vi "SO2 TCP Packet_v3.vi"(7 "TCP Packet In":string, 13 "Data Array":string[](array[string])) -> (8 "TCP Binary Packet":string)   [LabVIEW 2014]
panel:
  out "array":string[](array[string])
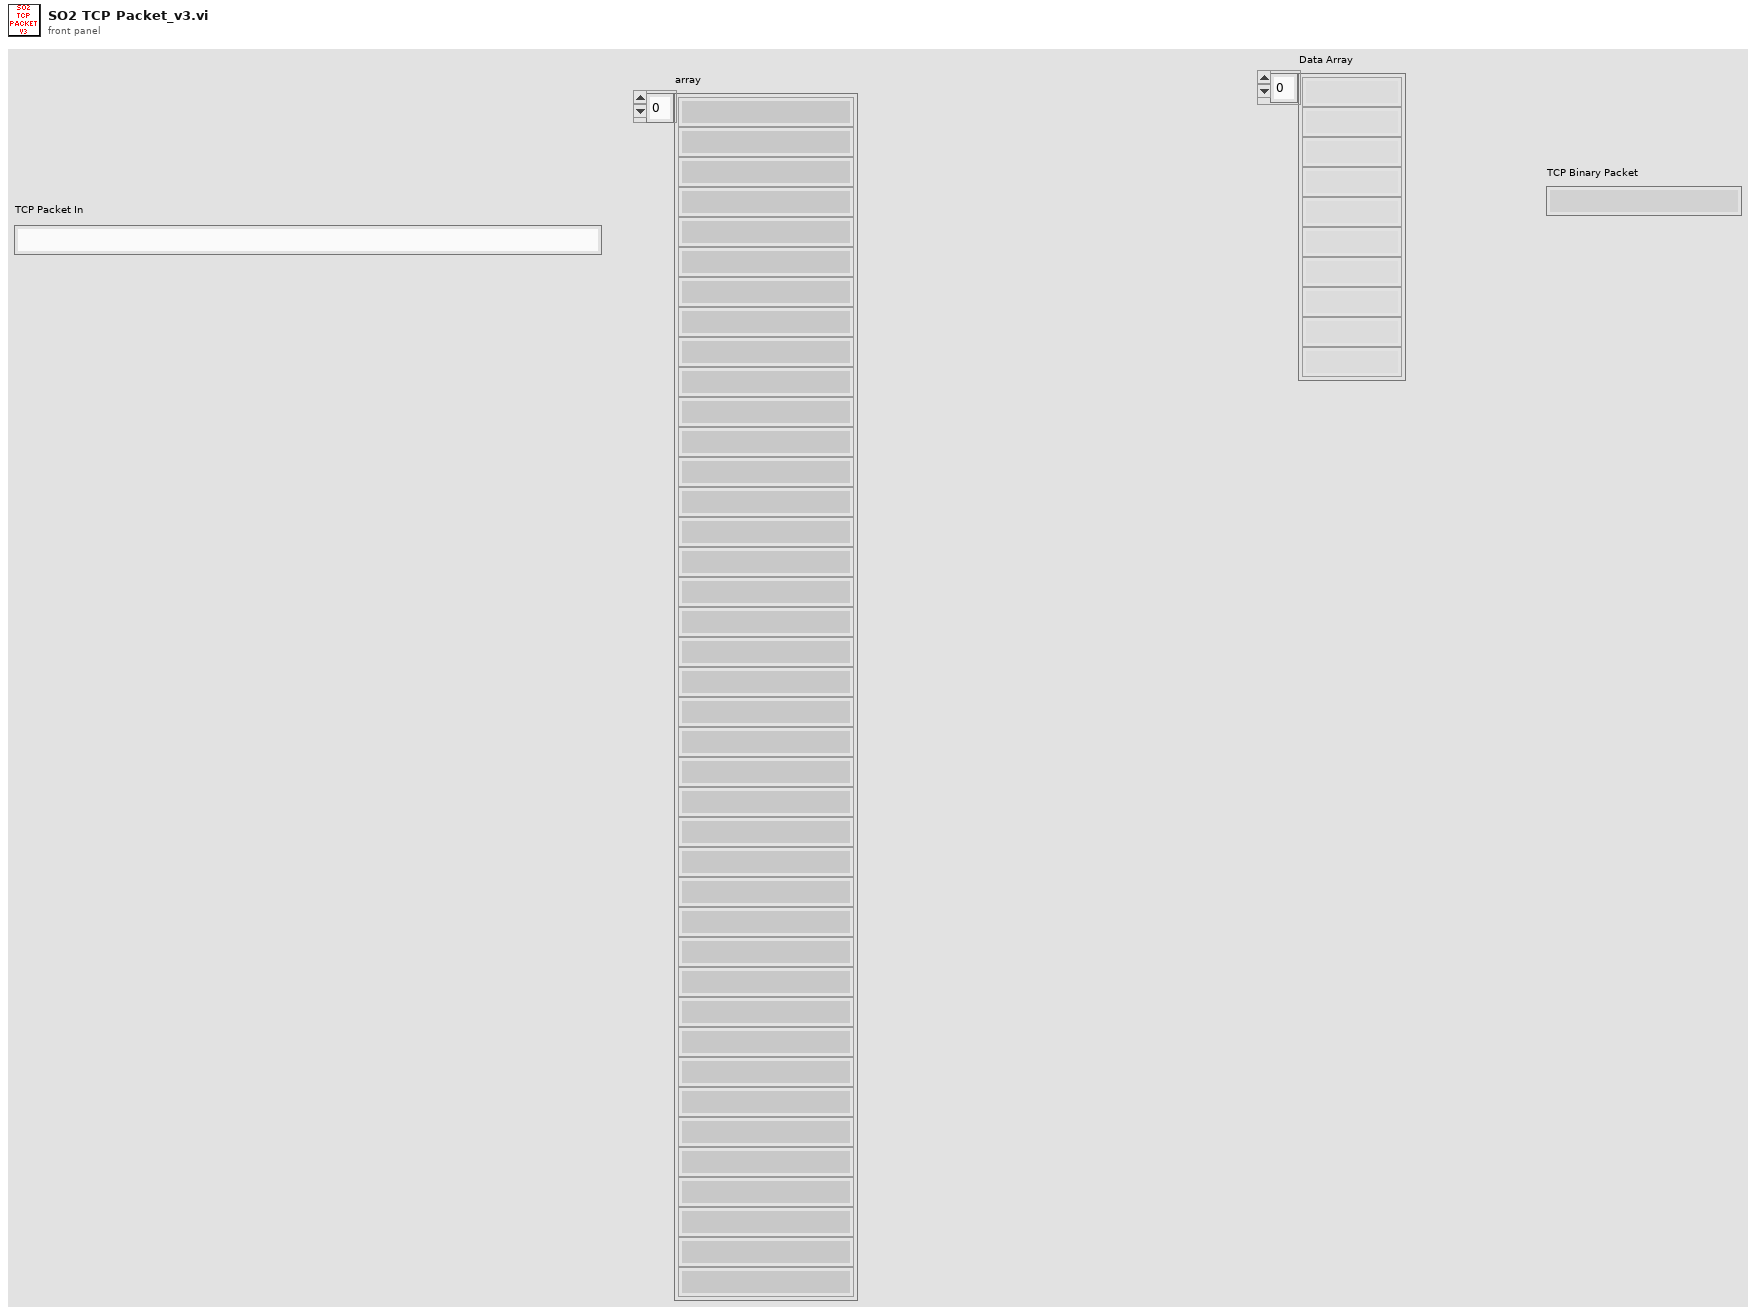
[diagram p1: front panel]
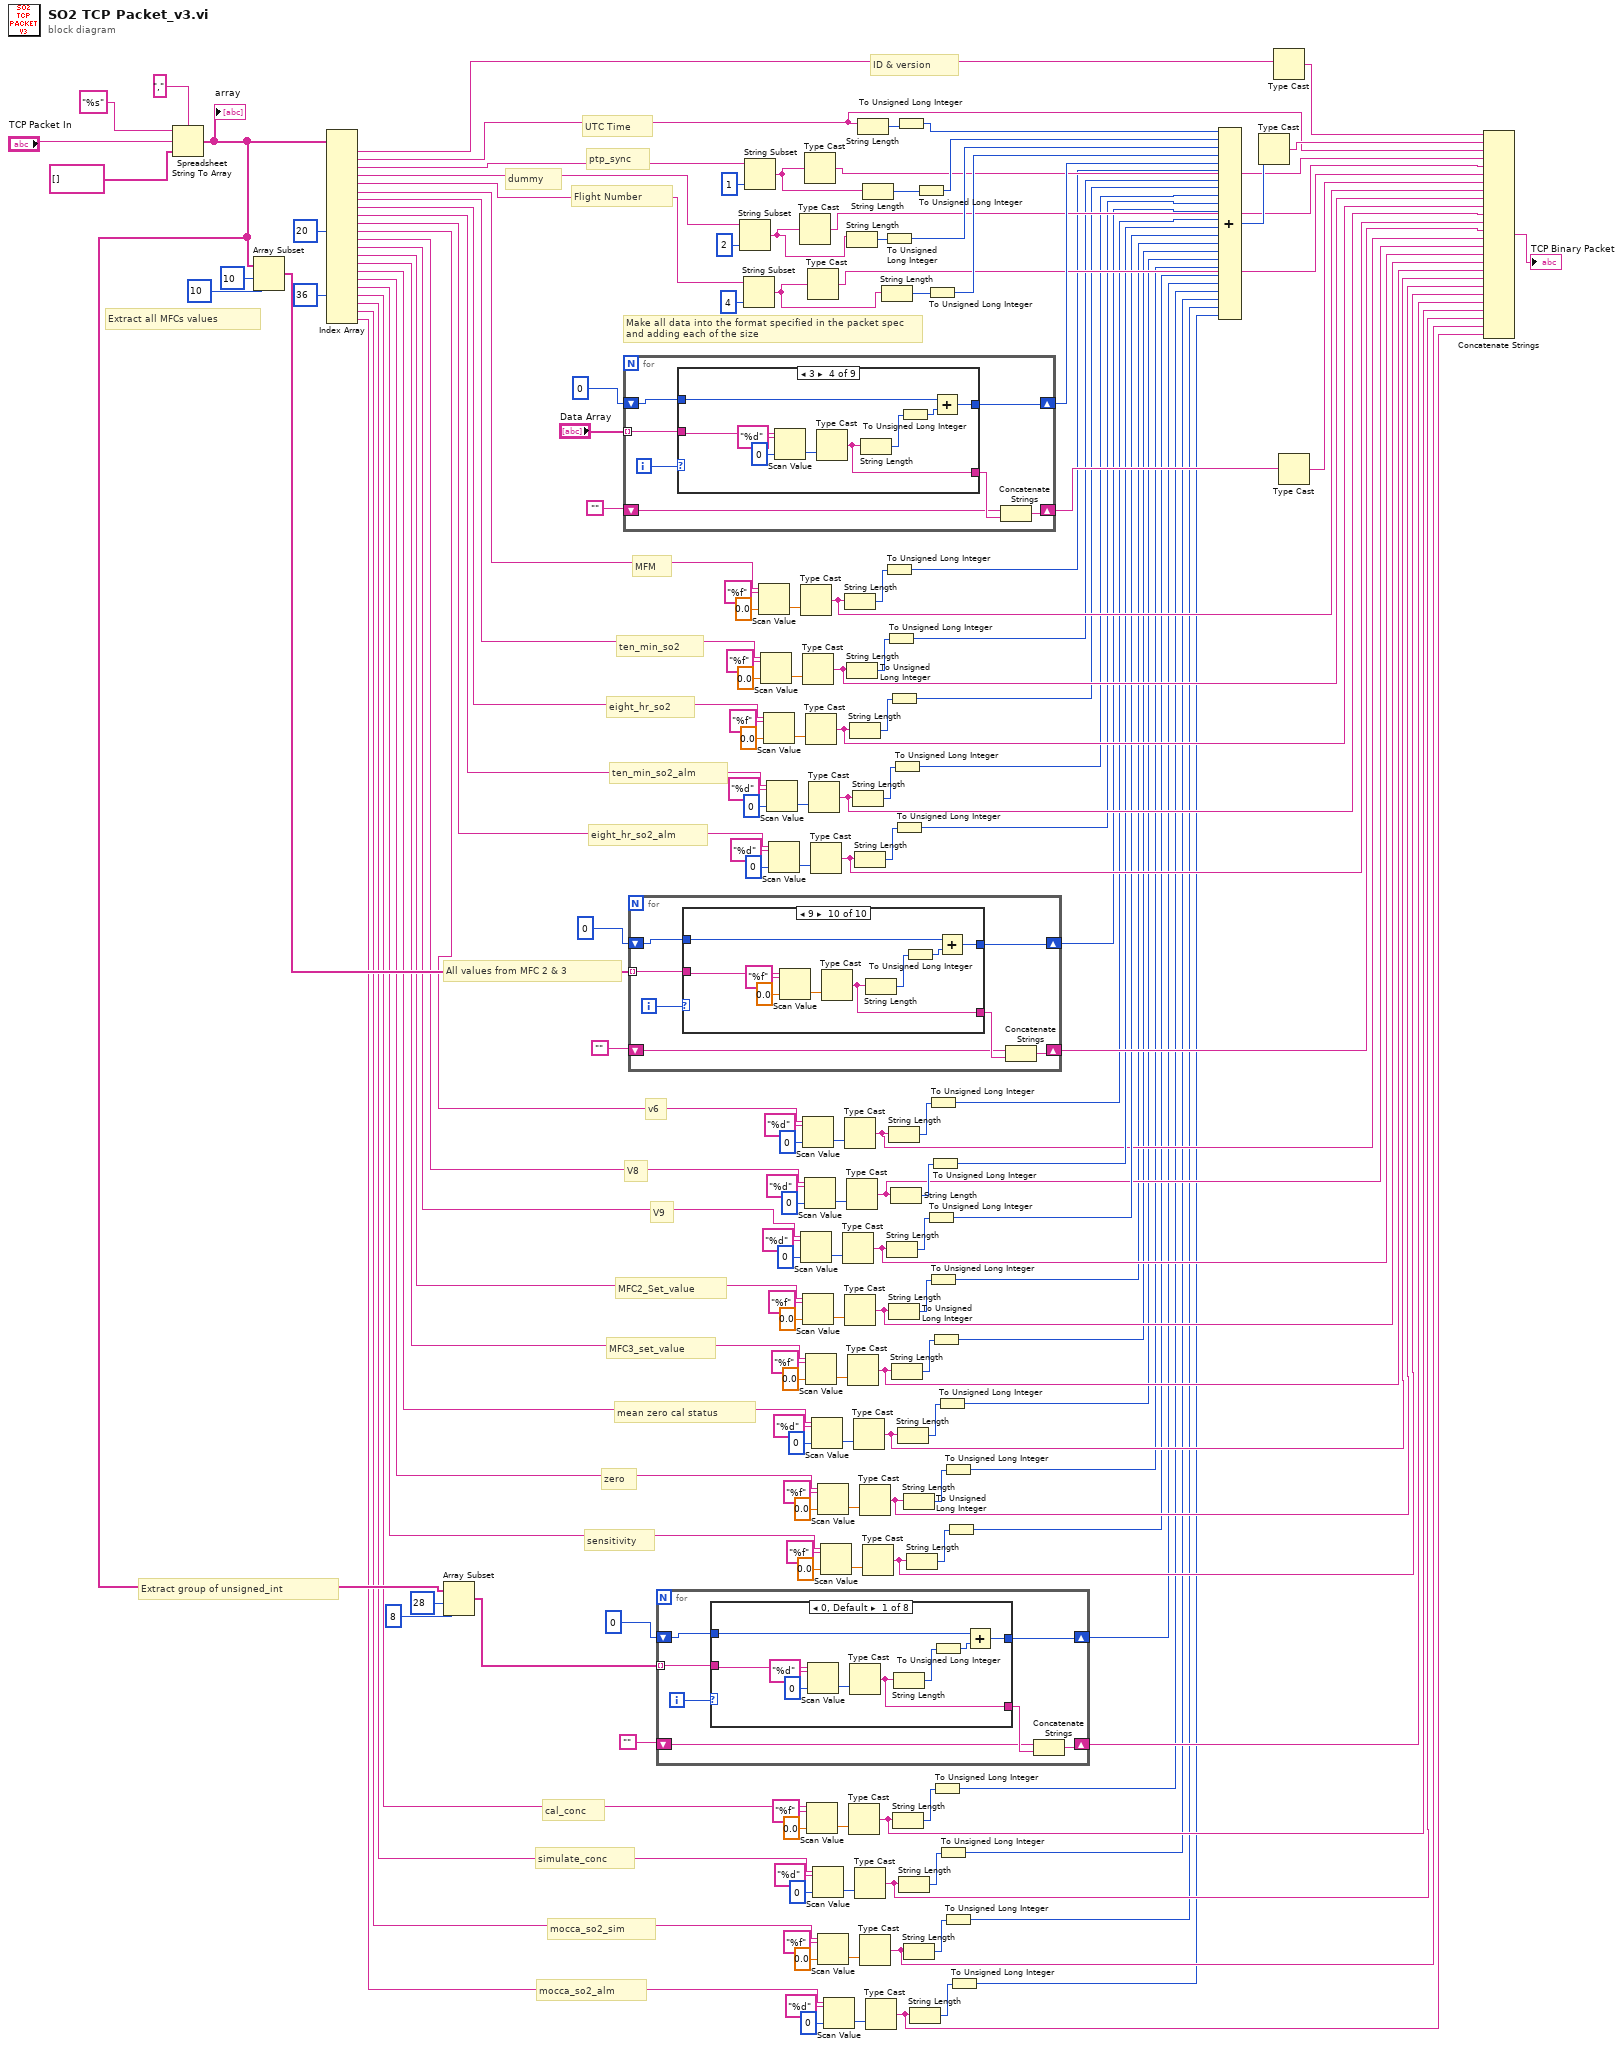
[diagram p0: block diagram]
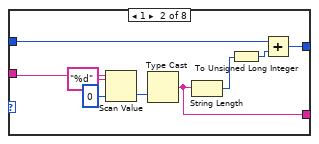
[diagram p2: hidden frame]
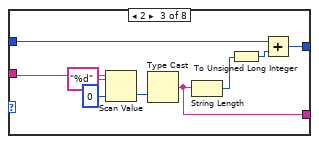
[diagram p3: hidden frame]
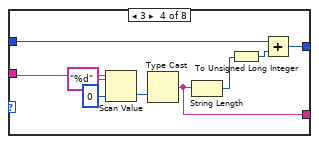
[diagram p4: hidden frame]
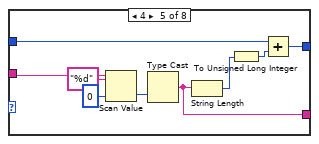
[diagram p5: hidden frame]
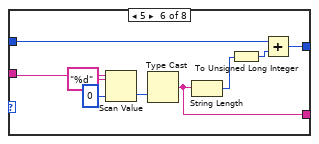
[diagram p6: hidden frame]
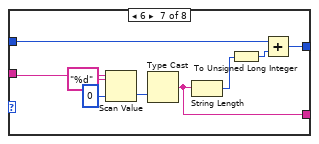
[diagram p7: hidden frame]
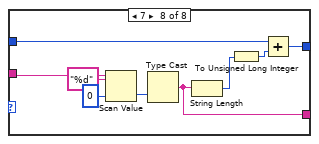
[diagram p8: hidden frame]
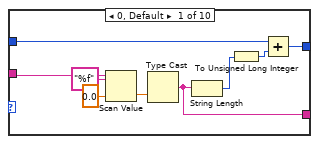
[diagram p9: hidden frame]
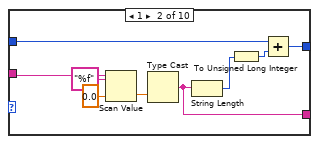
[diagram p10: hidden frame]
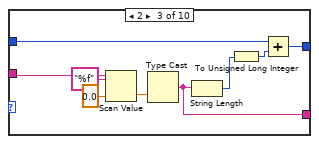
[diagram p11: hidden frame]
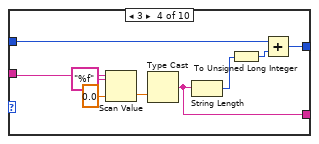
[diagram p12: hidden frame]
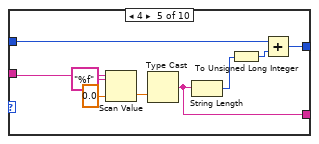
[diagram p13: hidden frame]
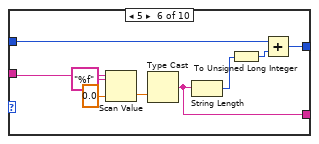
[diagram p14: hidden frame]
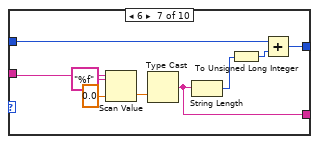
[diagram p15: hidden frame]
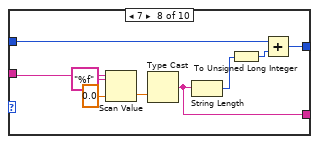
[diagram p16: hidden frame]
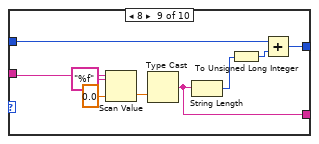
[diagram p17: hidden frame]
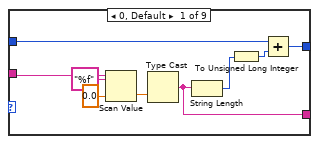
[diagram p18: hidden frame]
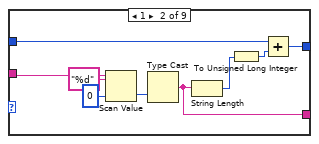
[diagram p19: hidden frame]
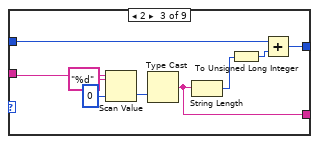
[diagram p20: hidden frame]
diagram:
  # "mocca_so2_alm"
  # "mocca_so2_sim"
  # "simulate_conc"
  # "cal_conc"
  # "Extract group of unsigned_int"
  # "sensitivity"
  # "zero"
  # "mean zero cal status"
  # "MFC3_set_value"
  # "MFC2_Set_value"
  # "V9"
  # "V8"
  # "v6"
  # "All values from MFC 2 & 3"
  # "Extract all MFCs values"
  # "eight_hr_so2_alm"
  # "ten_min_so2_alm"
  # "eight_hr_so2"
  # "ten_min_so2"
  # "MFM"
  # "Flight Number"
  # "dummy"
  # "ptp_sync"
  # "UTC Time"
  # "ID & version"
  # "Make all data into the format specified in the packet spec\nand adding each of the size"
  n1 = Spreadsheet String To Array(delimiter (Tab)=",", format string="%s", spreadsheet string="TCP Packet In", array type (2D Dbl)=string[] []) -> (array=w35:string[])
  "array" <- w35
  n2 = Array Subset(array=w35, index=10, length=10) -> (w97:string[])
  n3 = Index Array(array=w35, index #11=20 ("index"), index #19=36 ("index")) -> (element #1=w141:string, element #2=w140:string, element #3=w139:string, element #4=w138:string, element #5=w137:string, element #6=w132:string, element #7=w121:string, element #8=w118:string, element #9=w107:string, element #10=w104:string, element #11=w85:string, element #12=w84:string, element #13=w79:string, element #14=w64:string, element #15=w59:string, element #16=w54:string, element #17=w43:string, element #18=w38:string, element #19=w12:string, element #20=w3:string, element #21=w2:string, element #22=w1:string)  [unwired: 20 in]
  n4 = Array Subset(array=w35, index=28, length=8) -> (w31:string[])
  n5 = for {
    tunnel: "Data Array" -> [w178] mode=indexing
    shift-right: [w176] -> w160
    shift-left: u32 0 -> [w177]
    shift-right: [w175] -> w149
    shift-left: "" -> [w173]
    i -> [w179]
    n6 = case shown="3" w179 {
      tunnel: w178 -> [w186 w195 w204 w213 w222 w231 w240 w249 w253]
      tunnel: w177 -> [w184 w193 w202 w211 w220 w229 w238 w247 w259]
      tunnel: [w181 w190 w199 w208 w217 w226 w235 w244 w256] -> w176
      tunnel: [w180 w189 w198 w207 w216 w225 w234 w243 w255] -> w174
      frame 0, Default {
        n7 = Scan Value(string=w186, format string="%f", default (0 dbl)=sgl 0.0 ("default (0 I32)")) -> (value=w188:sgl)  [unwired: 1 out]
        n8 = Type Cast(x=w188) -> (*(type *) &x=w180:string)  [unwired: 1 in]
        n9 = String Length(string=w180) -> (length=w183:i32)
        n10 = To Unsigned Long Integer(number=w183) -> (unsigned 32bit integer=w182:u32)
        n11 = Add(x=w184, y=w182) -> (x+y=w181:u32)
      }
      frame 1 {
        n12 = Scan Value(string=w195, format string="%d", default (0 dbl)=0 ("default (0 I32)")) -> (value=w197:i32)  [unwired: 1 out]
        n13 = Type Cast(x=w197) -> (*(type *) &x=w189:string)  [unwired: 1 in]
        n14 = String Length(string=w189) -> (length=w192:i32)
        n15 = To Unsigned Long Integer(number=w192) -> (unsigned 32bit integer=w191:u32)
        n16 = Add(x=w193, y=w191) -> (x+y=w190:u32)
      }
      frame 2 {
        n17 = Scan Value(string=w204, format string="%d", default (0 dbl)=0 ("default (0 I32)")) -> (value=w206:i32)  [unwired: 1 out]
        n18 = Type Cast(x=w206) -> (*(type *) &x=w198:string)  [unwired: 1 in]
        n19 = String Length(string=w198) -> (length=w201:i32)
        n20 = To Unsigned Long Integer(number=w201) -> (unsigned 32bit integer=w200:u32)
        n21 = Add(x=w202, y=w200) -> (x+y=w199:u32)
      }
      frame 3 {
        n22 = Scan Value(string=w213, format string="%d", default (0 dbl)=0 ("default (0 I32)")) -> (value=w215:i32)  [unwired: 1 out]
        n23 = Type Cast(x=w215) -> (*(type *) &x=w207:string)  [unwired: 1 in]
        n24 = String Length(string=w207) -> (length=w210:i32)
        n25 = To Unsigned Long Integer(number=w210) -> (unsigned 32bit integer=w209:u32)
        n26 = Add(x=w211, y=w209) -> (x+y=w208:u32)
      }
      frame 4 {
        n27 = Scan Value(string=w222, format string="%f", default (0 dbl)=sgl 0.0 ("default (0 I32)")) -> (value=w224:sgl)  [unwired: 1 out]
        n28 = Type Cast(x=w224) -> (*(type *) &x=w216:string)  [unwired: 1 in]
        n29 = String Length(string=w216) -> (length=w219:i32)
        n30 = To Unsigned Long Integer(number=w219) -> (unsigned 32bit integer=w218:u32)
        n31 = Add(x=w220, y=w218) -> (x+y=w217:u32)
      }
      frame 5 {
        n32 = Scan Value(string=w231, format string="%f", default (0 dbl)=sgl 0.0 ("default (0 I32)")) -> (value=w233:sgl)  [unwired: 1 out]
        n33 = Type Cast(x=w233) -> (*(type *) &x=w225:string)  [unwired: 1 in]
        n34 = String Length(string=w225) -> (length=w228:i32)
        n35 = To Unsigned Long Integer(number=w228) -> (unsigned 32bit integer=w227:u32)
        n36 = Add(x=w229, y=w227) -> (x+y=w226:u32)
      }
      frame 6 {
        n37 = Scan Value(string=w240, format string="%f", default (0 dbl)=sgl 0.0 ("default (0 I32)")) -> (value=w242:sgl)  [unwired: 1 out]
        n38 = Type Cast(x=w242) -> (*(type *) &x=w234:string)  [unwired: 1 in]
        n39 = String Length(string=w234) -> (length=w237:i32)
        n40 = To Unsigned Long Integer(number=w237) -> (unsigned 32bit integer=w236:u32)
        n41 = Add(x=w238, y=w236) -> (x+y=w235:u32)
      }
      frame 7 {
        n42 = Scan Value(string=w249, format string="%f", default (0 dbl)=sgl 0.0 ("default (0 I32)")) -> (value=w251:sgl)  [unwired: 1 out]
        n43 = Type Cast(x=w251) -> (*(type *) &x=w243:string)  [unwired: 1 in]
        n44 = String Length(string=w243) -> (length=w246:i32)
        n45 = To Unsigned Long Integer(number=w246) -> (unsigned 32bit integer=w245:u32)
        n46 = Add(x=w247, y=w245) -> (x+y=w244:u32)
      }
      frame 8 {
        n47 = String Subset(string=w253, length (rest)=8 ("length (rest)")) -> (substring=w252:string)  [unwired: 1 in]
        n48 = Type Cast(x=w252) -> (*(type *) &x=w255:string)  [unwired: 1 in]
        n49 = String Length(string=w255) -> (length=w258:i32)
        n50 = To Unsigned Long Integer(number=w258) -> (unsigned 32bit integer=w257:u32)
        n51 = Add(x=w259, y=w257) -> (x+y=w256:u32)
      }
    }
    n52 = Concatenate Strings(w173, w174) -> (w175:string)
  }
  n53 = for {
    tunnel: w97 -> [w265] mode=indexing
    shift-right: [w263] -> w96
    shift-left: u32 0 -> [w264]
    shift-right: [w262] -> w95
    shift-left: "" -> [w260]
    i -> [w266]
    n54 = case shown="9" w266 {
      tunnel: w265 -> [w273 w282 w291 w300 w309 w318 w327 w336 w345 w354]
      tunnel: w264 -> [w271 w280 w289 w298 w307 w316 w325 w334 w343 w352]
      tunnel: [w268 w277 w286 w295 w304 w313 w322 w331 w340 w349] -> w263
      tunnel: [w267 w276 w285 w294 w303 w312 w321 w330 w339 w348] -> w261
      frame 0, Default {
        n55 = Scan Value(string=w273, format string="%f", default (0 dbl)=sgl 0.0 ("default (0 I32)")) -> (value=w275:sgl)  [unwired: 1 out]
        n56 = Type Cast(x=w275) -> (*(type *) &x=w267:string)  [unwired: 1 in]
        n57 = String Length(string=w267) -> (length=w270:i32)
        n58 = To Unsigned Long Integer(number=w270) -> (unsigned 32bit integer=w269:u32)
        n59 = Add(x=w271, y=w269) -> (x+y=w268:u32)
      }
      frame 1 {
        n60 = Scan Value(string=w282, format string="%f", default (0 dbl)=sgl 0.0 ("default (0 I32)")) -> (value=w284:sgl)  [unwired: 1 out]
        n61 = Type Cast(x=w284) -> (*(type *) &x=w276:string)  [unwired: 1 in]
        n62 = String Length(string=w276) -> (length=w279:i32)
        n63 = To Unsigned Long Integer(number=w279) -> (unsigned 32bit integer=w278:u32)
        n64 = Add(x=w280, y=w278) -> (x+y=w277:u32)
      }
      frame 2 {
        n65 = Scan Value(string=w291, format string="%f", default (0 dbl)=sgl 0.0 ("default (0 I32)")) -> (value=w293:sgl)  [unwired: 1 out]
        n66 = Type Cast(x=w293) -> (*(type *) &x=w285:string)  [unwired: 1 in]
        n67 = String Length(string=w285) -> (length=w288:i32)
        n68 = To Unsigned Long Integer(number=w288) -> (unsigned 32bit integer=w287:u32)
        n69 = Add(x=w289, y=w287) -> (x+y=w286:u32)
      }
      frame 3 {
        n70 = Scan Value(string=w300, format string="%f", default (0 dbl)=sgl 0.0 ("default (0 I32)")) -> (value=w302:sgl)  [unwired: 1 out]
        n71 = Type Cast(x=w302) -> (*(type *) &x=w294:string)  [unwired: 1 in]
        n72 = String Length(string=w294) -> (length=w297:i32)
        n73 = To Unsigned Long Integer(number=w297) -> (unsigned 32bit integer=w296:u32)
        n74 = Add(x=w298, y=w296) -> (x+y=w295:u32)
      }
      frame 4 {
        n75 = Scan Value(string=w309, format string="%f", default (0 dbl)=sgl 0.0 ("default (0 I32)")) -> (value=w311:sgl)  [unwired: 1 out]
        n76 = Type Cast(x=w311) -> (*(type *) &x=w303:string)  [unwired: 1 in]
        n77 = String Length(string=w303) -> (length=w306:i32)
        n78 = To Unsigned Long Integer(number=w306) -> (unsigned 32bit integer=w305:u32)
        n79 = Add(x=w307, y=w305) -> (x+y=w304:u32)
      }
      frame 5 {
        n80 = Scan Value(string=w318, format string="%f", default (0 dbl)=sgl 0.0 ("default (0 I32)")) -> (value=w320:sgl)  [unwired: 1 out]
        n81 = Type Cast(x=w320) -> (*(type *) &x=w312:string)  [unwired: 1 in]
        n82 = String Length(string=w312) -> (length=w315:i32)
        n83 = To Unsigned Long Integer(number=w315) -> (unsigned 32bit integer=w314:u32)
        n84 = Add(x=w316, y=w314) -> (x+y=w313:u32)
      }
      frame 6 {
        n85 = Scan Value(string=w327, format string="%f", default (0 dbl)=sgl 0.0 ("default (0 I32)")) -> (value=w329:sgl)  [unwired: 1 out]
        n86 = Type Cast(x=w329) -> (*(type *) &x=w321:string)  [unwired: 1 in]
        n87 = String Length(string=w321) -> (length=w324:i32)
        n88 = To Unsigned Long Integer(number=w324) -> (unsigned 32bit integer=w323:u32)
        n89 = Add(x=w325, y=w323) -> (x+y=w322:u32)
      }
      frame 7 {
        n90 = Scan Value(string=w336, format string="%f", default (0 dbl)=sgl 0.0 ("default (0 I32)")) -> (value=w338:sgl)  [unwired: 1 out]
        n91 = Type Cast(x=w338) -> (*(type *) &x=w330:string)  [unwired: 1 in]
        n92 = String Length(string=w330) -> (length=w333:i32)
        n93 = To Unsigned Long Integer(number=w333) -> (unsigned 32bit integer=w332:u32)
        n94 = Add(x=w334, y=w332) -> (x+y=w331:u32)
      }
      frame 8 {
        n95 = Scan Value(string=w345, format string="%f", default (0 dbl)=sgl 0.0 ("default (0 I32)")) -> (value=w347:sgl)  [unwired: 1 out]
        n96 = Type Cast(x=w347) -> (*(type *) &x=w339:string)  [unwired: 1 in]
        n97 = String Length(string=w339) -> (length=w342:i32)
        n98 = To Unsigned Long Integer(number=w342) -> (unsigned 32bit integer=w341:u32)
        n99 = Add(x=w343, y=w341) -> (x+y=w340:u32)
      }
      frame 9 {
        n100 = Scan Value(string=w354, format string="%f", default (0 dbl)=sgl 0.0 ("default (0 I32)")) -> (value=w356:sgl)  [unwired: 1 out]
        n101 = Type Cast(x=w356) -> (*(type *) &x=w348:string)  [unwired: 1 in]
        n102 = String Length(string=w348) -> (length=w351:i32)
        n103 = To Unsigned Long Integer(number=w351) -> (unsigned 32bit integer=w350:u32)
        n104 = Add(x=w352, y=w350) -> (x+y=w349:u32)
      }
    }
    n105 = Concatenate Strings(w260, w261) -> (w262:string)
  }
  n106 = for {
    tunnel: w31 -> [w362] mode=indexing
    shift-right: [w360] -> w30
    shift-left: u32 0 -> [w361]
    shift-right: [w359] -> w29
    shift-left: "" -> [w357]
    i -> [w363]
    n107 = case shown="0, Default" w363 {
      tunnel: w362 -> [w370 w379 w388 w397 w406 w415 w424 w433]
      tunnel: w361 -> [w368 w377 w386 w395 w404 w413 w422 w431]
      tunnel: [w365 w374 w383 w392 w401 w410 w419 w428] -> w360
      tunnel: [w364 w373 w382 w391 w400 w409 w418 w427] -> w358
      frame 0, Default {
        n108 = Scan Value(string=w370, format string="%d", default (0 dbl)=u16 0 ("default (0 I32)")) -> (value=w372:u16)  [unwired: 1 out]
        n109 = Type Cast(x=w372) -> (*(type *) &x=w364:string)  [unwired: 1 in]
        n110 = String Length(string=w364) -> (length=w367:i32)
        n111 = To Unsigned Long Integer(number=w367) -> (unsigned 32bit integer=w366:u32)
        n112 = Add(x=w368, y=w366) -> (x+y=w365:u32)
      }
      frame 1 {
        n113 = Scan Value(string=w379, format string="%d", default (0 dbl)=u16 0 ("default (0 I32)")) -> (value=w381:u16)  [unwired: 1 out]
        n114 = Type Cast(x=w381) -> (*(type *) &x=w373:string)  [unwired: 1 in]
        n115 = String Length(string=w373) -> (length=w376:i32)
        n116 = To Unsigned Long Integer(number=w376) -> (unsigned 32bit integer=w375:u32)
        n117 = Add(x=w377, y=w375) -> (x+y=w374:u32)
      }
      frame 2 {
        n118 = Scan Value(string=w388, format string="%d", default (0 dbl)=u16 0 ("default (0 I32)")) -> (value=w390:u16)  [unwired: 1 out]
        n119 = Type Cast(x=w390) -> (*(type *) &x=w382:string)  [unwired: 1 in]
        n120 = String Length(string=w382) -> (length=w385:i32)
        n121 = To Unsigned Long Integer(number=w385) -> (unsigned 32bit integer=w384:u32)
        n122 = Add(x=w386, y=w384) -> (x+y=w383:u32)
      }
      frame 3 {
        n123 = Scan Value(string=w397, format string="%d", default (0 dbl)=u16 0 ("default (0 I32)")) -> (value=w399:u16)  [unwired: 1 out]
        n124 = Type Cast(x=w399) -> (*(type *) &x=w391:string)  [unwired: 1 in]
        n125 = String Length(string=w391) -> (length=w394:i32)
        n126 = To Unsigned Long Integer(number=w394) -> (unsigned 32bit integer=w393:u32)
        n127 = Add(x=w395, y=w393) -> (x+y=w392:u32)
      }
      frame 4 {
        n128 = Scan Value(string=w406, format string="%d", default (0 dbl)=u16 0 ("default (0 I32)")) -> (value=w408:u16)  [unwired: 1 out]
        n129 = Type Cast(x=w408) -> (*(type *) &x=w400:string)  [unwired: 1 in]
        n130 = String Length(string=w400) -> (length=w403:i32)
        n131 = To Unsigned Long Integer(number=w403) -> (unsigned 32bit integer=w402:u32)
        n132 = Add(x=w404, y=w402) -> (x+y=w401:u32)
      }
      frame 5 {
        n133 = Scan Value(string=w415, format string="%d", default (0 dbl)=u16 0 ("default (0 I32)")) -> (value=w417:u16)  [unwired: 1 out]
        n134 = Type Cast(x=w417) -> (*(type *) &x=w409:string)  [unwired: 1 in]
        n135 = String Length(string=w409) -> (length=w412:i32)
        n136 = To Unsigned Long Integer(number=w412) -> (unsigned 32bit integer=w411:u32)
        n137 = Add(x=w413, y=w411) -> (x+y=w410:u32)
      }
      frame 6 {
        n138 = Scan Value(string=w424, format string="%d", default (0 dbl)=u16 0 ("default (0 I32)")) -> (value=w426:u16)  [unwired: 1 out]
        n139 = Type Cast(x=w426) -> (*(type *) &x=w418:string)  [unwired: 1 in]
        n140 = String Length(string=w418) -> (length=w421:i32)
        n141 = To Unsigned Long Integer(number=w421) -> (unsigned 32bit integer=w420:u32)
        n142 = Add(x=w422, y=w420) -> (x+y=w419:u32)
      }
      frame 7 {
        n143 = Scan Value(string=w433, format string="%d", default (0 dbl)=u16 0 ("default (0 I32)")) -> (value=w435:u16)  [unwired: 1 out]
        n144 = Type Cast(x=w435) -> (*(type *) &x=w427:string)  [unwired: 1 in]
        n145 = String Length(string=w427) -> (length=w430:i32)
        n146 = To Unsigned Long Integer(number=w430) -> (unsigned 32bit integer=w429:u32)
        n147 = Add(x=w431, y=w429) -> (x+y=w428:u32)
      }
    }
    n148 = Concatenate Strings(w357, w358) -> (w359:string)
  }
  n149 = String Subset(string=w138, length (rest)=2 ("length (rest)")) -> (substring=w147:string)  [unwired: 1 in]
  n150 = String Subset(string=w137, length (rest)=4 ("length (rest)")) -> (substring=w153:string)  [unwired: 1 in]
  n151 = String Subset(string=w139, length (rest)=1 ("length (rest)")) -> (substring=w156:string)  [unwired: 1 in]
  n152 = Scan Value(string=w132, format string="%f", default (0 dbl)=sgl 0.0 ("default (0 I32)")) -> (value=w136:sgl)  [unwired: 1 out]
  n153 = Scan Value(string=w121, format string="%f", default (0 dbl)=sgl 0.0 ("default (0 I32)")) -> (value=w129:sgl)  [unwired: 1 out]
  n154 = Scan Value(string=w118, format string="%f", default (0 dbl)=sgl 0.0 ("default (0 I32)")) -> (value=w125:sgl)  [unwired: 1 out]
  n155 = Scan Value(string=w107, format string="%d", default (0 dbl)=u16 0 ("default (0 I32)")) -> (value=w115:u16)  [unwired: 1 out]
  n156 = Scan Value(string=w104, format string="%d", default (0 dbl)=u16 0 ("default (0 I32)")) -> (value=w111:u16)  [unwired: 1 out]
  n157 = Type Cast(x=w147) -> (*(type *) &x=w146:string)  [unwired: 1 in]
  n158 = Type Cast(x=w136) -> (*(type *) &x=w130:string)  [unwired: 1 in]
  n159 = Scan Value(string=w79, format string="%d", default (0 dbl)=u16 0 ("default (0 I32)")) -> (value=w83:u16)  [unwired: 1 out]
  n160 = Type Cast(x=w129) -> (*(type *) &x=w119:string)  [unwired: 1 in]
  n161 = Scan Value(string=w85, format string="%d", default (0 dbl)=u16 0 ("default (0 I32)")) -> (value=w93:u16)  [unwired: 1 out]
  n162 = Scan Value(string=w64, format string="%f", default (0 dbl)=sgl 0.0 ("default (0 I32)")) -> (value=w72:sgl)  [unwired: 1 out]
  n163 = Type Cast(x=w156) -> (*(type *) &x=w155:string)  [unwired: 1 in]
  n164 = Scan Value(string=w84, format string="%d", default (0 dbl)=u16 0 ("default (0 I32)")) -> (value=w89:u16)  [unwired: 1 out]
  n165 = Type Cast(x=w125) -> (*(type *) &x=w116:string)  [unwired: 1 in]
  n166 = Scan Value(string=w59, format string="%f", default (0 dbl)=sgl 0.0 ("default (0 I32)")) -> (value=w68:sgl)  [unwired: 1 out]
  n167 = Scan Value(string=w12, format string="%f", default (0 dbl)=sgl 0.0 ("default (0 I32)")) -> (value=w28:sgl)  [unwired: 1 out]
  n168 = Type Cast(x=w153) -> (*(type *) &x=w154:string)  [unwired: 1 in]
  n169 = Type Cast(x=w115) -> (*(type *) &x=w105:string)  [unwired: 1 in]
  n170 = Type Cast(x=w111) -> (*(type *) &x=w102:string)  [unwired: 1 in]
  n171 = Scan Value(string=w54, format string="%d", default (0 dbl)=u16 0 ("default (0 I32)")) -> (value=w58:u16)  [unwired: 1 out]
  n172 = Scan Value(string=w3, format string="%d", default (0 dbl)=u16 0 ("default (0 I32)")) -> (value=w24:u16)  [unwired: 1 out]
  n173 = Scan Value(string=w43, format string="%f", default (0 dbl)=sgl 0.0 ("default (0 I32)")) -> (value=w51:sgl)  [unwired: 1 out]
  n174 = Scan Value(string=w2, format string="%f", default (0 dbl)=sgl 0.0 ("default (0 I32)")) -> (value=w20:sgl)  [unwired: 1 out]
  n175 = Scan Value(string=w38, format string="%f", default (0 dbl)=sgl 0.0 ("default (0 I32)")) -> (value=w47:sgl)  [unwired: 1 out]
  n176 = Scan Value(string=w1, format string="%d", default (0 dbl)=u16 0 ("default (0 I32)")) -> (value=w16:u16)  [unwired: 1 out]
  n177 = Type Cast(x=w83) -> (*(type *) &x=w73:string)  [unwired: 1 in]
  n178 = String Length(string=w130) -> (length=w133:i32)
  n179 = Type Cast(x=w93) -> (*(type *) &x=w75:string)  [unwired: 1 in]
  n180 = Type Cast(x=w72) -> (*(type *) &x=w62:string)  [unwired: 1 in]
  n181 = String Length(string=w147) -> (length=w167:i32)
  n182 = String Length(string=w119) -> (length=w126:i32)
  n183 = Type Cast(x=w89) -> (*(type *) &x=w74:string)  [unwired: 1 in]
  n184 = Type Cast(x=w68) -> (*(type *) &x=w60:string)  [unwired: 1 in]
  n185 = Type Cast(x=w28) -> (*(type *) &x=w10:string)  [unwired: 1 in]
  n186 = String Length(string=w116) -> (length=w122:i32)
  n187 = String Length(string=w105) -> (length=w112:i32)
  n188 = Type Cast(x=w58) -> (*(type *) &x=w52:string)  [unwired: 1 in]
  n189 = String Length(string=w102) -> (length=w108:i32)
  n190 = Type Cast(x=w24) -> (*(type *) &x=w8:string)  [unwired: 1 in]
  n191 = String Length(string=w140) -> (length=w172:i32)
  n192 = Type Cast(x=w51) -> (*(type *) &x=w41:string)  [unwired: 1 in]
  n193 = Type Cast(x=w20) -> (*(type *) &x=w6:string)  [unwired: 1 in]
  n194 = String Length(string=w156) -> (length=w169:i32)
  n195 = Type Cast(x=w47) -> (*(type *) &x=w39:string)  [unwired: 1 in]
  n196 = Type Cast(x=w16) -> (*(type *) &x=w4:string)  [unwired: 1 in]
  n197 = String Length(string=w153) -> (length=w164:i32)
  n198 = To Unsigned Long Integer(number=w167) -> (unsigned 32bit integer=w166:u32)
  n199 = To Unsigned Long Integer(number=w133) -> (unsigned 32bit integer=w131:u32)
  n200 = To Unsigned Long Integer(number=w126) -> (unsigned 32bit integer=w120:u32)
  n201 = String Length(string=w73) -> (length=w80:i32)
  n202 = To Unsigned Long Integer(number=w122) -> (unsigned 32bit integer=w117:u32)
  n203 = String Length(string=w75) -> (length=w90:i32)
  n204 = String Length(string=w62) -> (length=w69:i32)
  n205 = String Length(string=w74) -> (length=w86:i32)
  n206 = To Unsigned Long Integer(number=w112) -> (unsigned 32bit integer=w106:u32)
  n207 = String Length(string=w60) -> (length=w65:i32)
  n208 = String Length(string=w10) -> (length=w25:i32)
  n209 = To Unsigned Long Integer(number=w108) -> (unsigned 32bit integer=w103:u32)
  n210 = To Unsigned Long Integer(number=w172) -> (unsigned 32bit integer=w171:u32)
  n211 = String Length(string=w52) -> (length=w55:i32)
  n212 = String Length(string=w8) -> (length=w21:i32)
  n213 = String Length(string=w41) -> (length=w48:i32)
  n214 = String Length(string=w6) -> (length=w17:i32)
  n215 = String Length(string=w39) -> (length=w44:i32)
  n216 = String Length(string=w4) -> (length=w13:i32)
  n217 = To Unsigned Long Integer(number=w169) -> (unsigned 32bit integer=w168:u32)
  n218 = To Unsigned Long Integer(number=w80) -> (unsigned 32bit integer=w76:u32)
  n219 = To Unsigned Long Integer(number=w164) -> (unsigned 32bit integer=w163:u32)
  n220 = To Unsigned Long Integer(number=w90) -> (unsigned 32bit integer=w78:u32)
  n221 = To Unsigned Long Integer(number=w69) -> (unsigned 32bit integer=w63:u32)
  n222 = To Unsigned Long Integer(number=w86) -> (unsigned 32bit integer=w77:u32)
  n223 = To Unsigned Long Integer(number=w65) -> (unsigned 32bit integer=w61:u32)
  n224 = To Unsigned Long Integer(number=w25) -> (unsigned 32bit integer=w11:u32)
  n225 = To Unsigned Long Integer(number=w55) -> (unsigned 32bit integer=w53:u32)
  n226 = To Unsigned Long Integer(number=w21) -> (unsigned 32bit integer=w9:u32)
  n227 = To Unsigned Long Integer(number=w48) -> (unsigned 32bit integer=w42:u32)
  n228 = To Unsigned Long Integer(number=w17) -> (unsigned 32bit integer=w7:u32)
  n229 = To Unsigned Long Integer(number=w44) -> (unsigned 32bit integer=w40:u32)
  n230 = To Unsigned Long Integer(number=w13) -> (unsigned 32bit integer=w5:u32)
  n231 = Compound Arithmetic op=ADD(w171, w168, w166, w163, w160, w131, w120, w117, w106, w103, w96, w78, w77, w76, w63, w61, w53, w42, w40, w30, w11, w9, w7, w5) -> (w158:u32)
  n232 = Type Cast(x=w158) -> (*(type *) &x=w157:string)  [unwired: 1 in]
  n233 = Type Cast(x=w141) -> (*(type *) &x=w159:string)  [unwired: 1 in]
  n234 = Type Cast(x=w149) -> (*(type *) &x=w152:string)  [unwired: 1 in]
  n235 = Concatenate Strings(w159, w157, w140, w155, w146, w154, w152, w130, w119, w116, w105, w102, w95, w75, w74, w73, w62, w60, w52, w41, w39, w29, w10, w8, w6, w4) -> (→"TCP Binary Packet":string)
